vi "数值到十六进制字符串.vi"(10 "Numeric":u32=23, 11 "转换字节数":enum16{"1字节", "2字节", "4字节", "3字节"}(ring)) -> (2 "二字节互换":string, 3 "转换结果":string)   [LabVIEW 2013]
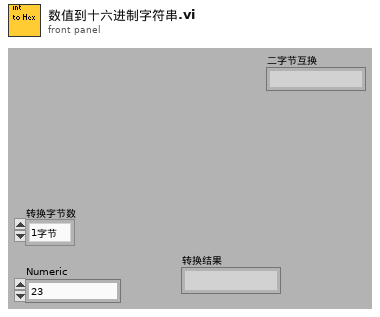
[diagram p1: front panel]
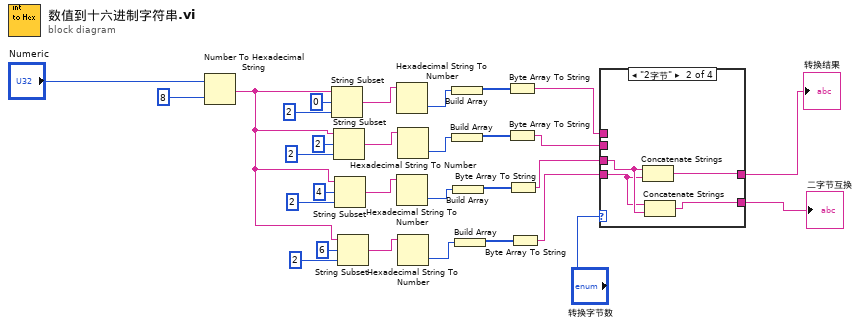
[diagram p0: block diagram]
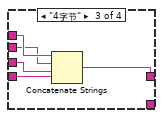
[diagram p3: hidden frame]
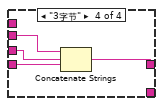
[diagram p4: hidden frame]
diagram:
  n1 = Number To Hexadecimal String(1:i16 8 ("width (-)"), 2:"Numeric") -> (0:w21:string)
  n2 = String Subset(string=w21, offset (0)=0, length (rest)=2 ("length (rest)")) -> (substring=w20:string)
  n3 = String Subset(string=w21, offset (0)=2, length (rest)=2 ("length (rest)")) -> (substring=w19:string)
  n4 = String Subset(string=w21, offset (0)=4, length (rest)=2 ("length (rest)")) -> (substring=w18:string)
  n5 = String Subset(string=w21, offset (0)=6, length (rest)=2 ("length (rest)")) -> (substring=w17:string)
  n6 = Hexadecimal String To Number(string=w20) -> (number=w12:u32)  [unwired: 3 out]
  n7 = Hexadecimal String To Number(string=w18) -> (number=w10:u32)  [unwired: 3 out]
  n8 = Hexadecimal String To Number(string=w19) -> (number=w11:u32)  [unwired: 3 out]
  n9 = Hexadecimal String To Number(string=w17) -> (number=w9:u32)  [unwired: 3 out]
  n10 = Build Array(w12) -> (w16:u32[])
  n11 = Build Array(w11) -> (w15:u32[])
  n12 = Build Array(w10) -> (w14:u32[])
  n13 = Build Array(w9) -> (w13:u32[])
  n14 = Byte Array To String(unsigned byte array=w16) -> (string=w2:string)
  n15 = Byte Array To String(unsigned byte array=w15) -> (string=w3:string)
  n16 = Byte Array To String(unsigned byte array=w14) -> (string=w4:string)
  n17 = Byte Array To String(unsigned byte array=w13) -> (string=w5:string)
  n18 = case shown="\"2字节\"" "转换字节数" {
    tunnel: [w31 w35 w38 w42] -> w6
    tunnel: w5 -> [w31 w33 w40 w44]
    tunnel: w4 -> [_ w34 w39 w43]
    tunnel: w3 -> [_ _ w36 w41]
    tunnel: w2 -> [_ _ w37 _]
    tunnel: [_ w32 _ _] -> w1
    frame "1字节", Default {
    }
    frame "2字节" {
      n19 = Concatenate Strings(w34, w33) -> (w35:string)
      n20 = Concatenate Strings(w33, w34) -> (w32:string)
    }
    frame "4字节" {
      n21 = Concatenate Strings(w37, w36, w39, w40) -> (w38:string)
    }
    frame "3字节" {
      n22 = Concatenate Strings(w41, w43, w44) -> (w42:string)
    }
  }
  "转换结果" <- w6
  "二字节互换" <- w1
